vi "Login to stop exe.vi"(8 "error in (no error) 2":errorcluster) -> (2 "error in (no error)":errorcluster, 3 "Success":bool)   [LabVIEW 2017]
panel:
  in  "OK Button":bool
  in  "Password":string
  # "Enter password to stop program"
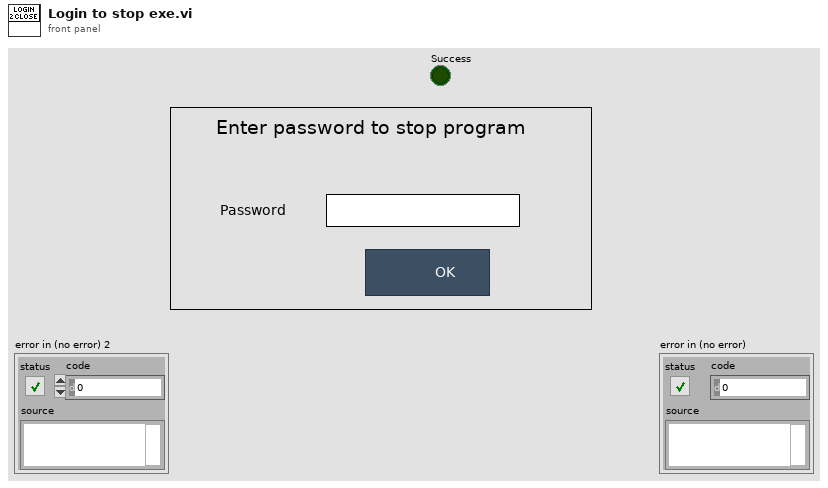
[diagram p1: front panel]
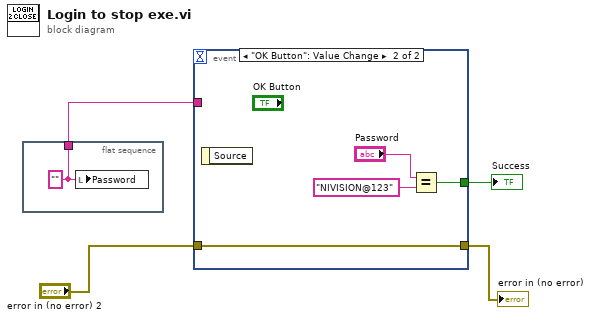
[diagram p0: block diagram]
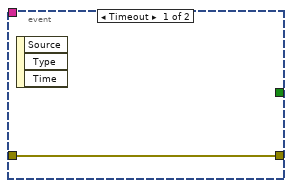
[diagram p2: hidden frame]
diagram:
  n1 = flat-sequence {
    tunnel: [w5] -> w3
    frame #0 {
      w5 = "" ("Password")
      n2 = local write "Password"(w5) -> ()
    }
  }
  n3 = event shown="[1] \"OK Button\": Value Change" {
    selector: _ -> [_ _]
    dyn-events: _ -> [_ _]
    timeout: _ -> [_ _]
    tunnel: [_ w8] -> w4
    tunnel: w3 -> [_ _]
    tunnel: "error in (no error) 2" -> [w6 w7]
    tunnel: [w6 w7] -> w1
    event Timeout {
      n4 = event-data() -> ()  [unwired: 1 in, 3 out]
    }
    event "OK Button": Value Change {
      n5 = event-data() -> ()  [unwired: 1 in, 1 out]
      n6 = Equal?(x="Password", y="NIVISION@123") -> (x = y?=w8:bool)
    }
  }
  "Success" <- w4
  "error in (no error)" <- w1
